vi "read_write.vi"() -> ()   [LabVIEW 2017]
uses:
  <userlib>/dxl_x86_c/dxl_x86_c.lvlib
panel:
  out "dynamixel_comm_result":string
  out "dynamixel_error":string
  in  "device_name":string="COM3"
  in  "ADDR_MX_\nPRESENT_POSITION":u16=36
  in  "ADDR_MX_\nGOAL_POSITION":u16=30
  in  "ADDR_MX_\nTORQUE_ENABLE":u16=24
  out "protocol_version":dbl=1.0
  out "value : MX (knob)\npresent position":u16(knob)=3387
  in  "terminate":bool
  out "port_num":i32
  in  "value : MX (dial)\ngoal position":u16(knob)=1979
  in  "dynamixel_id":u8=1
  in  "baud_rate":i32=57600
  # "/*******************************************************************************\n* Copyright (c) 2016, ROBOTIS CO., LTD.\n* All rights reserved.\n*\n* Redistribution and use in source and binary forms, with or without\n* modification, are permitted provided that the following conditions are met:\n*\n* * Redistributions of source code must retain the above copyright notice, this\n*   list of conditions and the following disclaimer.\n*\n* * Redistributions in binary form must reproduce the above copyright notice,\n*   this list of conditions and the following disclaimer in the documentation\n*   and/or other materials provided with the distribution.\n*\n* * Neither the name of ROBOTIS nor the names of its\n*   contributors may be used to endorse or promote products derived from\n*   this software without specific prior written permission.\n*\n* THIS SOFTWARE IS PROVIDED BY THE COPYRIGHT HOLDERS AND CONTRIBUTORS \"AS IS\"\n* AND ANY EXPRESS OR IMPLIED WARRANTIES, INCLUDING, BUT NOT LIMITED TO, THE\n* IMPLIED WARRANTIES OF MERCHANTABILITY AND FITNESS FOR A PARTICULAR PURPOSE ARE\n* DISCLAIMED. IN NO EVENT SHALL THE COPYRIGHT HOLDER OR CONTRIBUTORS BE LIABLE\n* FOR ANY DIRECT, INDIRECT, INCIDENTAL, SPECIAL, EXEMPLARY, OR CONSEQUENTIAL\n* DAMAGES (INCLUDING, BUT NOT LIMITED TO, PROCUREMENT OF SUBSTITUTE GOODS OR\n* SERVICES; LOSS OF USE, DATA, OR PROFITS; OR BUSINESS INTERRUPTION) HOWEVER\n* CAUSED AND ON ANY THEORY OF LIABILITY, WHETHER IN CONTRACT, STRICT LIABILITY,\n* OR TORT (INCLUDING NEGLIGENCE OR OTHERWISE) ARISING IN ANY WAY OUT OF THE USE\n* OF THIS SOFTWARE, EVEN IF ADVISED OF THE POSSIBILITY OF SUCH DAMAGE.\n*******************************************************************************/\n\n/* Author: Ryu Woon Jung (Leon) */"
  # "Available Dynamixel model on this example : All models using Protocol 1.0\nThis example is designed for using a Dynamixel MX-28, and an USB2DYNAMIXEL.\nTo use another Dynamixel model, such as X series, see their details in E-Manual(support.robotis.com) \n   and edit \"numeric control\"s seen left with \"Edit Text\" tool.\nBe sure that Dynamixel MX properties are already set as %% ID : 1 / Baudnum : 34 (Baudrate : 57600)\n\n1. Run example by click above \"Run\" button (below \"Edit\" menu).\n2. Drag \"dial\" then you may see the Dynamixel and \"knob\" rotating\n3. To finish the example, press \"terminate\" button."
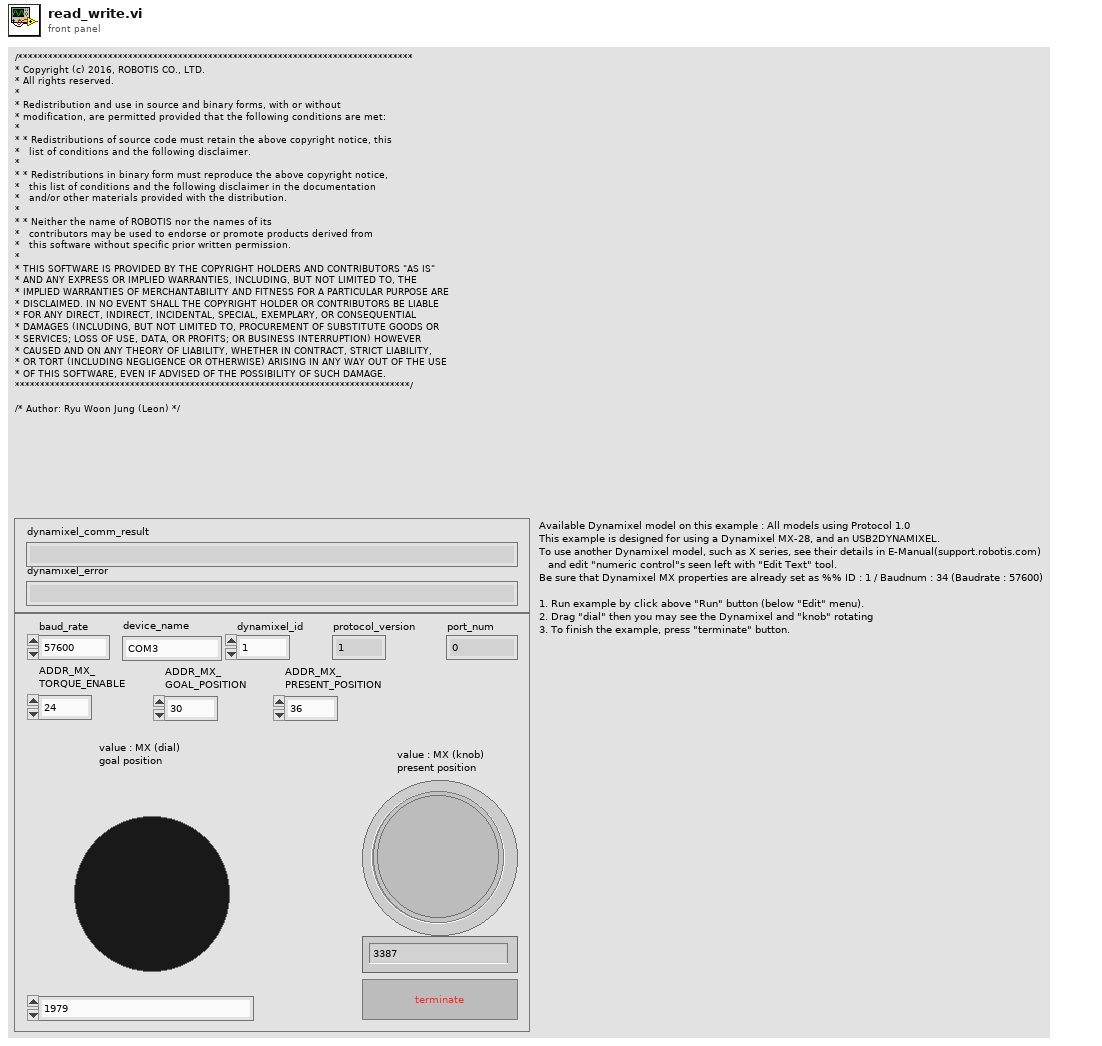
[diagram p1: front panel]
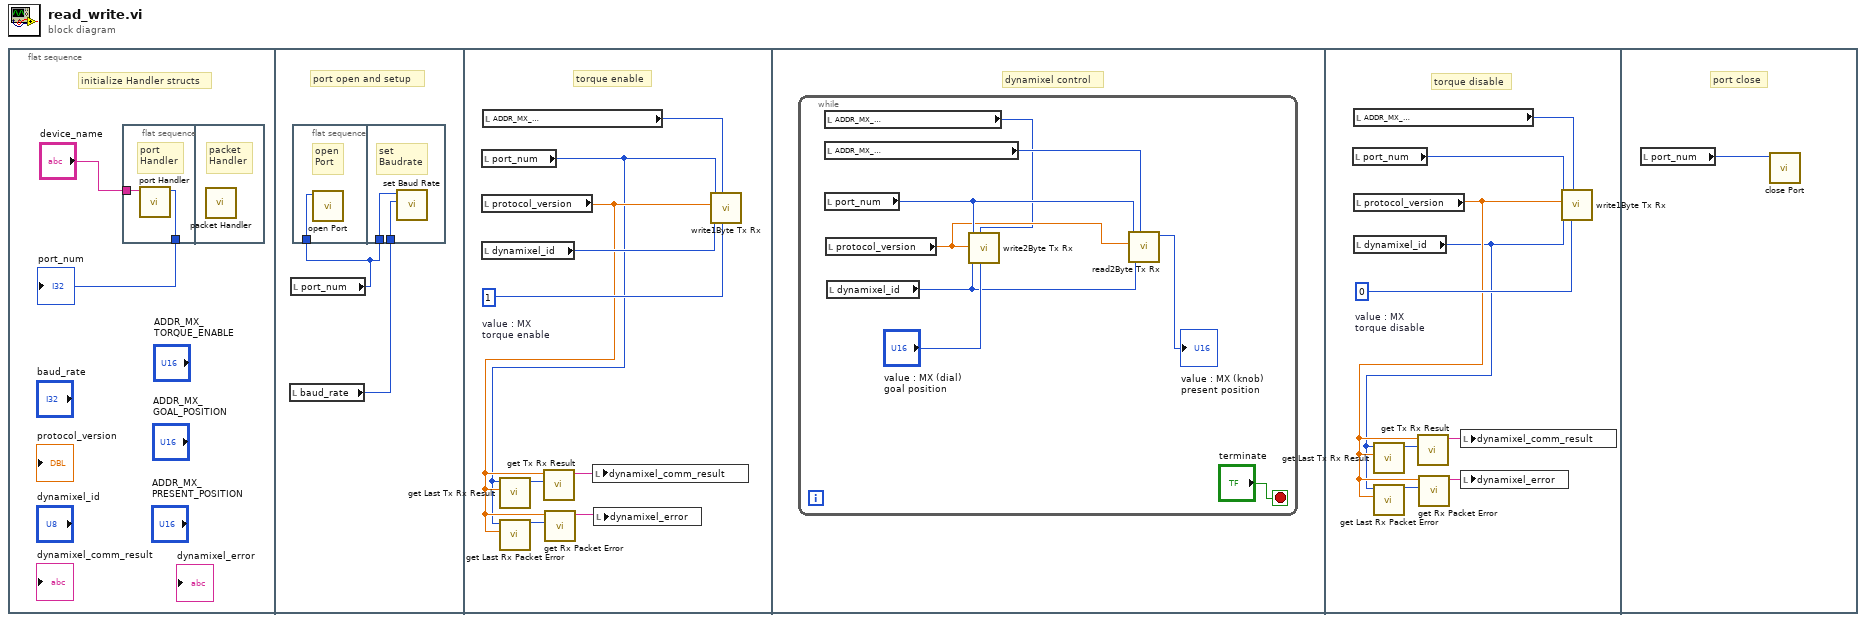
[diagram p0: block diagram]
diagram:
  n1 = flat-sequence {
    frame #0 {
      # "initialize Handler structs"
      n2 = flat-sequence {
        tunnel: [w4] -> w2
        tunnel: "device_name" -> [w3]
        frame #0 {
          # "port\nHandler"
          n3 = call <userlib>:"port Handler.vi"("port_name"=w3) -> ("function return"=w4:i32)  [unwired: 10 in]
        }
        frame #1 {
          # "packet\nHandler"
          n4 = call <userlib>:"packet Handler.vi"() -> ()  [unwired: 12 in]
        }
      }
      "port_num" <- w2
    }
    frame #1 {
      # "port open and setup"
      n5 = local read "baud_rate"() -> (w5:i32)
      n6 = local read "port_num"() -> (w6:i32)
      n7 = flat-sequence {
        tunnel: w6 -> [w7]
        tunnel: w6 -> [w9]
        tunnel: w5 -> [w8]
        frame #0 {
          # "open\nPort"
          n8 = call <userlib>:"open Port.vi"("port_num"=w7) -> ()  [unwired: 10 in, 1 out]
        }
        frame #1 {
          # "set\nBaudrate"
          n9 = call <userlib>:"set Baud Rate.vi"("baudrate"=w8, "port_num"=w9) -> ()  [unwired: 9 in, 1 out]
        }
      }
    }
    frame #2 {
      w18 = 1  # value : MX torque enable
      # "torque enable"
      n10 = local read "port_num"() -> (w10:i32)
      n11 = local read "protocol_version"() -> (w11:dbl)
      n12 = local read "dynamixel_id"() -> (w17:u8)
      n13 = local read "ADDR_MX_\nTORQUE_ENABLE"() -> (w16:u16)
      n14 = call <userlib>:"get Last Tx Rx Result.vi"("protocol_version"=w11, "port_num"=w10) -> ("function return"=w12:i32)  [unwired: 9 in]
      n15 = call <userlib>:"get Last Rx Packet Error.vi"("protocol_version"=w11, "port_num"=w10) -> ("function return"=w13:u8)  [unwired: 9 in]
      n16 = call <userlib>:"get Tx Rx Result.vi"("result"=w12, "protocol_version"=w11) -> ("function return"=w14:string)  [unwired: 9 in]
      n17 = call <userlib>:"get Rx Packet Error.vi"("error"=w13, "protocol_version"=w11) -> ("function return"=w15:string)  [unwired: 9 in]
      n18 = local write "dynamixel_comm_result"(w14) -> ()
      n19 = local write "dynamixel_error"(w15) -> ()
      n20 = call <userlib>:"write1Byte Tx Rx.vi"("data"=w18, "address"=w16, "id"=w17, "protocol_version"=w11, "port_num"=w10) -> ()  [unwired: 7 in]
    }
    frame #3 {
      # "dynamixel control"
      n21 = while {
        stop <- "terminate" stop-if-true
        n22 = local read "ADDR_MX_\nGOAL_POSITION"() -> (w19:u16)
        n23 = local read "ADDR_MX_\nPRESENT_POSITION"() -> (w20:u16)
        n24 = local read "port_num"() -> (w22:i32)
        n25 = local read "protocol_version"() -> (w21:dbl)
        n26 = local read "dynamixel_id"() -> (w23:u8)
        n27 = call <userlib>:"write2Byte Tx Rx.vi"("data"="value : MX (dial)\ngoal position", "address"=w19, "id"=w23, "protocol_version"=w21, "port_num"=w22) -> ()  [unwired: 7 in]
        n28 = call <userlib>:"read2Byte Tx Rx.vi"("address"=w20, "id"=w23, "protocol_version"=w21, "port_num"=w22) -> ("function return"=→"value : MX (knob)\npresent position":u16)  [unwired: 7 in]
      }
    }
    frame #4 {
      w34 = 0  # value : MX torque disable
      # "torque disable"
      n29 = local read "port_num"() -> (w35:i32)
      n30 = local read "ADDR_MX_\nTORQUE_ENABLE"() -> (w33:u16)
      n31 = local read "protocol_version"() -> (w28:dbl)
      n32 = local read "dynamixel_id"() -> (w27:u8)
      n33 = call <userlib>:"get Last Tx Rx Result.vi"("protocol_version"=w28, "port_num"=w27) -> ("function return"=w30:i32)  [unwired: 9 in]
      n34 = call <userlib>:"get Last Rx Packet Error.vi"("protocol_version"=w28, "port_num"=w27) -> ("function return"=w29:u8)  [unwired: 9 in]
      n35 = call <userlib>:"get Tx Rx Result.vi"("result"=w30, "protocol_version"=w28) -> ("function return"=w31:string)  [unwired: 9 in]
      n36 = call <userlib>:"get Rx Packet Error.vi"("error"=w29, "protocol_version"=w28) -> ("function return"=w32:string)  [unwired: 9 in]
      n37 = local write "dynamixel_comm_result"(w31) -> ()
      n38 = local write "dynamixel_error"(w32) -> ()
      n39 = call <userlib>:"write1Byte Tx Rx.vi"("data"=w34, "address"=w33, "id"=w27, "protocol_version"=w28, "port_num"=w35) -> ()  [unwired: 7 in]
    }
    frame #5 {
      # "port close"
      n40 = local read "port_num"() -> (w36:i32)
      n41 = call <userlib>:"close Port.vi"("port_num"=w36) -> ()  [unwired: 11 in]
    }
  }
